vi "Set ClusterArray Values from JSON String.vi"(8 "error in (no error)":errorcluster, 10 "Path to Settings JSON":path, 11 "Array in":refnum<vi>) -> (0 "error out":errorcluster)   [LabVIEW 2023]
panel:
  out "ClusterName out":string
  out "Outer Cluster":string
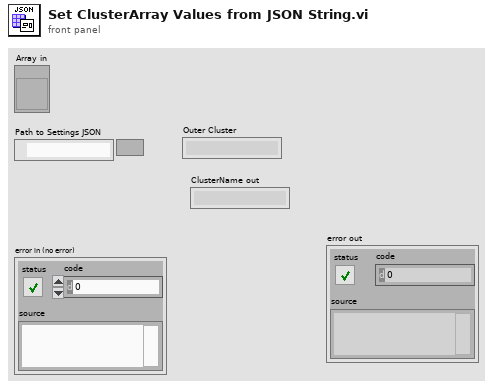
[diagram p1: front panel]
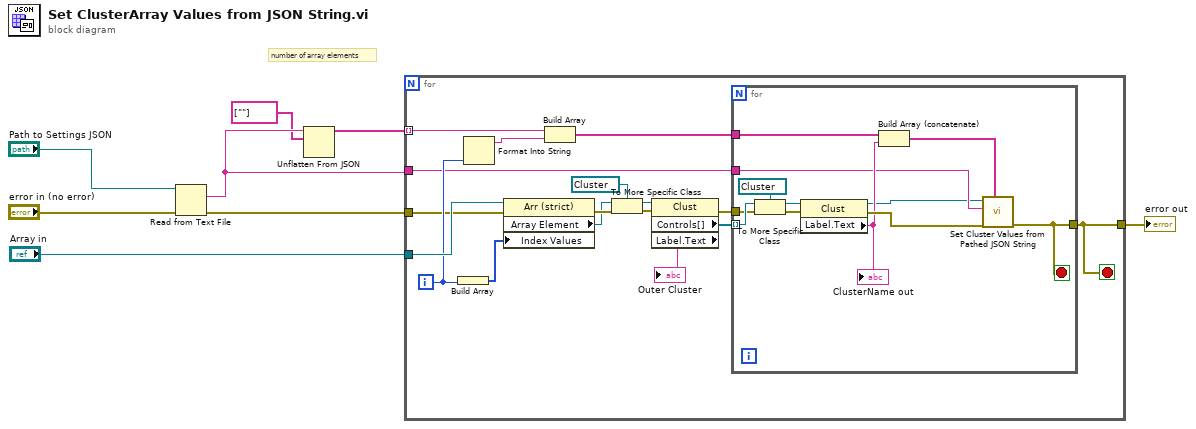
[diagram p0: block diagram]
diagram:
  # "number of array elements"
  n1 = Read from Text File(file (use dialog)="Path to Settings JSON", error in="error in (no error)") -> (text=w4:string, error out=w2:errorcluster)  [unwired: 2 in, 2 out]
  n2 = Unflatten From JSON(JSON string=w4, type and defaults=string[] [""]) -> (value=w7:string[])  [unwired: 5 in, 1 out]
  n3 = for {
    tunnel: w7 -> [w18] mode=indexing
    tunnel: "Array in" -> [w25]
    tunnel: [w23] -> w5
    tunnel: w4 -> [w9]
    tunnel: w2 -> [w21]
    i -> [w22]
    stop <- w23 stop-if-true
    n4 = Build Array(w22) -> (w24:i32[])
    n5 = Format Into String(w22) -> (resulting string=w19:string)  [unwired: 3 in, 1 out]
    n6 = property class="Arr (strict)"(reference=w25, error in=w21, "Index Values"=w24) -> (error out=w16:errorcluster, "Array Element"=w13:refnum<vi>)  [unwired: 1 out]
    n7 = Build Array(w18, w19) -> (w20:string[])
    n8 = To More Specific Class(target class=refnum<vi> refnum ("specific class reference"), reference=w13, error in=w16) -> (specific class reference=w14:refnum<vi>, error out=w15:errorcluster)
    n9 = property class="Clust"(reference=w14, error in=w15) -> (error out=w10:errorcluster, "Controls[]"=w12:refnum<vi>[], "Label.Text"=→"Outer Cluster":string)  [unwired: 1 out]
    n10 = for {
      tunnel: [w33] -> w23
      tunnel: w20 -> [w30]
      tunnel: w12 -> [w32] mode=indexing
      tunnel: w10 -> [w31]
      tunnel: w9 -> [w27]
      stop <- w33 stop-if-true
      n11 = To More Specific Class(target class=refnum<vi> refnum ("specific class reference"), reference=w32, error in=w31) -> (specific class reference=w37:refnum<vi>, error out=w36:errorcluster)
      n12 = property class="Clust"(reference=w37, error in=w36) -> (reference out=w26:refnum<vi>, error out=w35:errorcluster, "Label.Text"=w28:string)
      "ClusterName out" <- w28
      n13 = Build Array (concatenate)(w30, w28) -> (w29:string[])
      n14 = call "Set Cluster Values from Pathed JSON String.vi"("Path"=w29, "error in (no error)"=w35, "JSON string"=w27, "Clust Refnum"=w26) -> ("error out"=w33:errorcluster)  [unwired: 7 in]
    }
  }
  "error out" <- w5
